vi "6) HTTP Info.vi"() -> ()   [LabVIEW 2020, in "VectoScratch.lvlib"]
uses:
  VectoScratch.lvlib
  Vecto/Node Config/Node Config.lvclass
  Vecto/Vecto/Vecto.lvclass
  Vecto/VectoService/VectoInfo.lvclass
  Vecto/ChannelService/ChannelService.lvclass
  Vecto/Group Config/Group Config.lvclass
  Vecto/Group Info.ctl
  VectoConfig/VectoConfig.lvlib
  Vecto/RemoteDataService/RemoteDataService.lvclass
  Vecto/Group DBL/Group DBL.lvclass
  Vecto/Group Data Type.ctl
  C:/dev/lv20CE/relink/lv-vecto/Vecto/Group/Group.lvclass
  C:/dev/lv20CE/relink/lv-vecto/Vecto/Group DBL/Group DBL.lvclass
  Vecto/Group STR/Group STR.lvclass
  C:/dev/lv20CE/relink/lv-vecto/Vecto/Group STR/Group STR.lvclass
  Vecto/Node Config/Discovery Info.ctl
  Vecto/Node Config/Node Info.ctl
  Vecto/Node Config/HTTP Server Info.ctl
  Vecto/Channel Init.ctl
  Vecto/IP Resolver/IP Resolver.lvclass
  Vecto/Connection Type.ctl
  Vecto/Vecto.lvlib
  Vecto/Connection Info.ctl
  Vecto/Vecto Info.ctl
  Vecto/proto/ServiceType/Enumeration.ctl
  Vecto/proto/ServiceType/ServiceType.lvlib
  Vecto/proto/Service/Data.ctl
  Vecto/proto/Service/Service.lvlib
  Vecto/proto/Discovery/Data.ctl
  Vecto/proto/Discovery/Discovery.lvlib
  Vecto/Publish Config.ctl
panel:
  in  "Strings":string[](array[string])=["alpha", "beta", "gamma", "delta"]
  in  "Publish Config":T1={"Address"="239.0.0.101", "Port"=36987}
  in  "Values":dbl[](array[slide])=[0.0, 0.0, 0.0, 0.0, 0.0, 0.0] scale=0.0..100.0
  in  "Bind Address":string="192.168.42.59"
  in  "ID":u32=1
  in  "Start":bool
  out "Discovery":T2[](array[typedef]) {"ip" format="%.0x"}
  in  "Discovery Address":string="239.0.0.50"
  in  "Discovery Port":u16=36986
  out "Vecto Info":T5
  in  "stop":bool
  in  "Node Name":string="Alpha"
  in  "HTTP Port":u16=36987
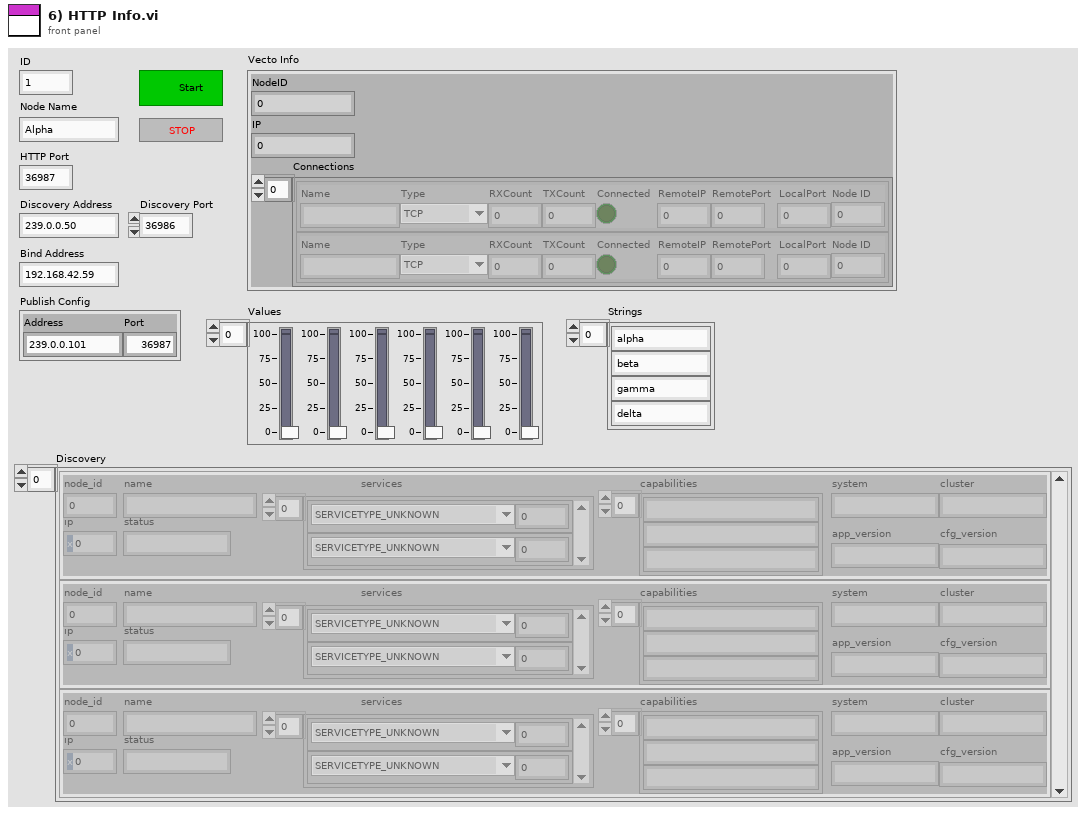
[diagram p1: front panel]
types:
  T1 = typedef "VectoConfig.lvlib/Publish Config.ctl" = cluster{"Address":string, "Port":u16}
  T2 = typedef "Discovery.lvlib/Data.ctl" = cluster{"node_id":u32, "name":string, "ip":u32, "status":string, "services":T3[], "capabilities":string[], "system":string, "cluster":string, "app_version":string, "cfg_version":string}
  T3 = typedef "Service.lvlib/Data.ctl" = cluster{"type":T4, "port":i32}
  T4 = typedef "ServiceType.lvlib/Enumeration.ctl" = enum16{"SERVICETYPE_UNKNOWN", "SERVICETYPE_TCPSERVER", "SERVICETYPE_HTTPSERVER"}
  T5 = typedef "Vecto.lvlib/Vecto Info.ctl" = cluster{"NodeID":i32, "IP":u32, "Connections":T6[]}
  T6 = typedef "Vecto.lvlib/Connection Info.ctl" = cluster{"Name":string, "Type":T7, "RXCount":i32, "TXCount":i32, "Connected":bool, "RemoteIP":u32, "RemotePort":u16, "LocalPort":u16, "Node ID":u32}
  T7 = typedef "Vecto.lvlib/Connection Type.ctl" = enum16{"TCP", "Telemetry", "Discovery", "HTTP"}
  T8 = typedef "VectoConfig.lvlib/Group Data Type.ctl" = enum16{"Double", "String", "Bool"}
  T9 = typedef "VectoConfig.lvlib/Group Info.ctl" = cluster{"System":string, "Cluster":string, "Node":string, "Task":string, "Name":string}
  T10 = typedef "VectoConfig.lvlib/HTTP Server Info.ctl" = cluster{"HTTP Port":u16, "Debug":bool}
  T11 = typedef "Discovery Info.ctl" = cluster{"Address":string, "Port":u16, "Interval S":dbl, "Bind Address":refnum<class "IP Resolver.lvclass">}
  T12 = typedef "VectoConfig.lvlib/Node Info.ctl" = cluster{"System":string, "Cluster":string, "Name":string, "ID":u32, "Capabilities":string[]}
  T13 = typedef "VectoConfig.lvlib/Channel Init.ctl" = cluster{"Name":string, "Resource":string, "Unit String":string}
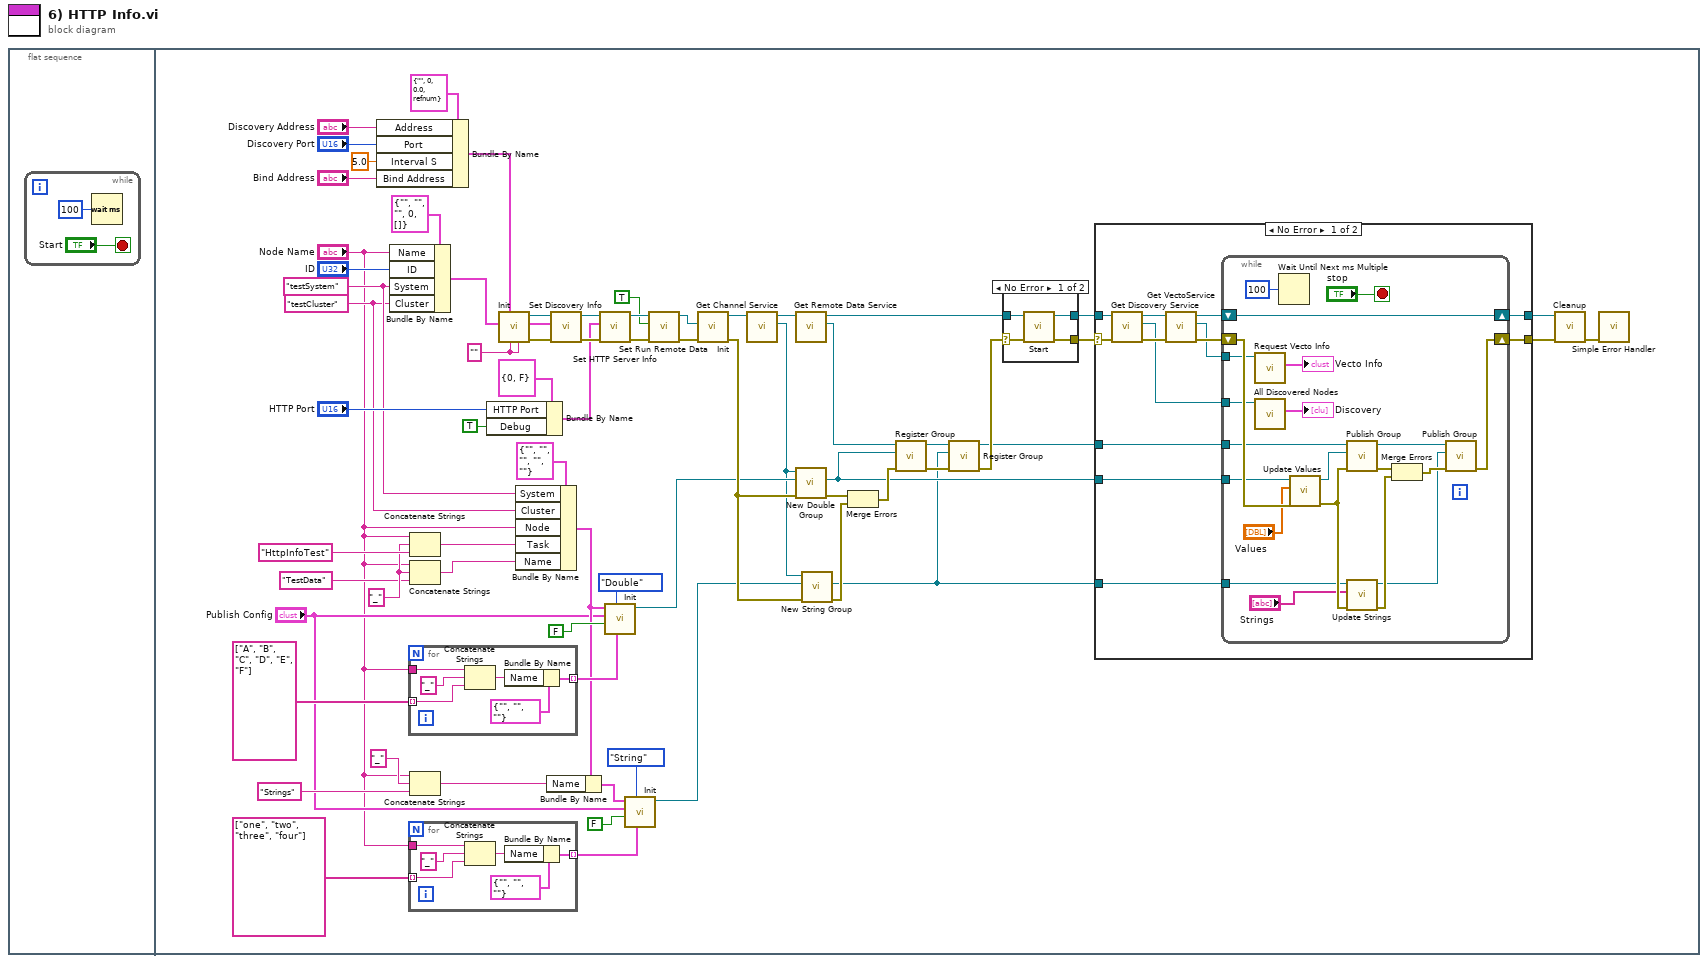
[diagram p0: block diagram]
diagram:
  n1 = flat-sequence {
    frame #0 {
      n2 = while {
        stop <- "Start" stop-if-true
        n3 = Wait (ms)(milliseconds to wait=u32 100) -> ()  [unwired: 1 out]
      }
    }
    frame #1 {
      w3 = "" ("Config Version")
      w30 = "_" ("string")
      w38 = "testCluster" ("System")
      w39 = "testSystem" ("System")
      n4 = Bundle By Name(cluster=T11 {"Address"="", "Port"=0, "Interval S"=0.0, "Bind Address"=refnum} ("Discovery Info"), "Address"="Discovery Address", "Port"="Discovery Port", "Interval S"=5.0, "Bind Address"="Bind Address") -> (w60:T11)
      n5 = Bundle By Name(cluster=T12 {"System"="", "Cluster"="", "Name"="", "ID"=0, "Capabilities"=[]} ("Node Info"), "Name"="Node Name", "ID"="ID", "System"=w39, "Cluster"=w38) -> (w56:T12)
      n6 = for {
        tunnel: string[] ["A", "B", "C", "D", "E", "F"] -> [w75] mode=indexing
        tunnel: "Node Name" -> [w74]
        tunnel: [w71] -> w26 mode=indexing
        n7 = Concatenate Strings(w74, "_" ("string"), w75) -> (w72:string)
        n8 = Bundle By Name(cluster=T13 {"Name"="", "Resource"="", "Unit String"=""} ("Channel Init"), "Name"=w72) -> (w71:T13)
      }
      n9 = for {
        tunnel: string[] ["one", "two", "three", "four"] -> [w123] mode=indexing
        tunnel: "Node Name" -> [w122]
        tunnel: [w119] -> w14 mode=indexing
        n10 = Concatenate Strings(w122, "_" ("string"), w123) -> (w120:string)
        n11 = Bundle By Name(cluster=T13 {"Name"="", "Resource"="", "Unit String"=""} ("Channel Init"), "Name"=w120) -> (w119:T13)
      }
      n12 = Concatenate Strings("Node Name", w30, "HttpInfoTest" ("Task")) -> (w31:string)
      n13 = Concatenate Strings("Node Name", w30, "TestData" ("Name")) -> (w28:string)
      n14 = Concatenate Strings("Node Name", "_" ("string"), "Strings" ("string")) -> (w21:string)
      n15 = Bundle By Name(cluster=T10 {"HTTP Port"=0, "Debug"=FALSE} ("HTTP Server Info"), "HTTP Port"="HTTP Port", "Debug"=TRUE) -> (w48:T10)
      n16 = call "Init.vi"("Config Hash"=w3, "Config Version"=w3, "Node Info"=w56) -> ("error out"=w63:errorcluster, "Node out"=w62:refnum<class "Node Config.lvclass">)  [unwired: 7 in]
      n17 = Bundle By Name(cluster=T9 {"System"="", "Cluster"="", "Node"="", "Task"="", "Name"=""} ("Group Info"), "System"=w39, "Cluster"=w38, "Node"="Node Name", "Task"=w31, "Name"=w28) -> (w24:T9)
      n18 = Bundle By Name(cluster=w24, "Name"=w21) -> (w20:T9)
      n19 = call "Set Discovery Info.vi"("error in (no error)"=w63, "Discovery Info"=w60, "Node in"=w62) -> ("error out"=w50:errorcluster, "Node out"=w51:refnum<class "Node Config.lvclass">)  [unwired: 7 in]
      n20 = call "Set HTTP Server Info.vi"("error in (no error)"=w50, "HTTP Server Info"=w48, "Node Config in"=w51) -> ("error out"=w45:errorcluster, "Node Config out"=w34:refnum<class "Node Config.lvclass">)  [unwired: 7 in]
      n21 = call "Init.vi"("Channels"=w26, "Group Data Type"=Group_Data_Type."Double", "Raw Values (T)"=FALSE, "Multicast Endpoint (None)"="Publish Config", "Group Info"=w24) -> ("Group Config out"=w42:refnum<class "Group Config.lvclass">)  [unwired: 5 in, 1 out]
      n22 = call "Init.vi"("Channels"=w14, "Group Data Type"=Group_Data_Type."String", "Raw Values (T)"=FALSE, "Multicast Endpoint (None)"="Publish Config", "Group Info"=w20) -> ("Group Config out"=w12:refnum<class "Group Config.lvclass">)  [unwired: 5 in, 1 out]
      n23 = call "Set Run Remote Data.vi"("error in (no error)"=w45, "Run Remote Data"=TRUE, "Node Config in"=w34) -> ("error out"=w35:errorcluster, "Node Config out"=w33:refnum<class "Node Config.lvclass">)  [unwired: 7 in]
      n24 = call "Init.vi"("error in (no error)"=w35, "Node"=w33) -> ("error out"=w70:errorcluster, "Vecto out"=w53:refnum<class "Vecto.lvclass">)  [unwired: 8 in]
      n25 = call "Get Channel Service.vi"("Vecto in"=w53) -> ("ChannelService"=w13:refnum<class "ChannelService.lvclass">, "Vecto out"=w52:refnum<class "Vecto.lvclass">)  [unwired: 8 in, 1 out]
      n26 = call "Get Remote Data Service.vi"("Vecto in"=w52) -> ("RemoteDataService"=w37:refnum<class "RemoteDataService.lvclass">, "Vecto out"=w44:refnum<class "Vecto.lvclass">)  [unwired: 8 in, 1 out]
      n27 = call "New Double Group.vi"("error in (no error)"=w70, "Group Config"=w42, "ChannelService in"=w13) -> ("error out"=w8:errorcluster, "Group"=w36:refnum<class "Group DBL.lvclass">)  [unwired: 6 in, 1 out]
      n28 = call "New String Group.vi"("error in (no error)"=w70, "Group Config"=w12, "ChannelService in"=w13) -> ("error out"=w69:errorcluster, "StringGroup"=w7:refnum<class "Group STR.lvclass">)  [unwired: 6 in, 1 out]
      n29 = Merge Errors(w8, w69) -> (w68:errorcluster)
      n30 = call "Register Group.vi"("error in (no error)"=w68, "Group"=w36, "RemoteDataService in"=w37) -> ("error out"=w67:errorcluster, "RemoteDataService out"=w11:refnum<class "RemoteDataService.lvclass">)  [unwired: 7 in]
      n31 = call "Register Group.vi"("error in (no error)"=w67, "Group"=w7, "RemoteDataService in"=w11) -> ("error out"=w10:errorcluster, "RemoteDataService out"=w9:refnum<class "RemoteDataService.lvclass">)  [unwired: 7 in]
      n32 = case shown="No Error" w10 {
        selector: w10 -> [w80 w82]
        tunnel: w44 -> [w79 w81]
        tunnel: [w78 w82] -> w66
        tunnel: [w77 w81] -> w65
        frame No Error {
          n33 = call "Start.vi"("error in (no error)"=w80, "Vecto in"=w79) -> ("error out"=w78:errorcluster, "Vecto out"=w77:refnum<class "Vecto.lvclass">)  [unwired: 8 in]
        }
        frame Error {
        }
      }
      n34 = case shown="No Error" w66 {
        selector: w66 -> [w91 w118]
        tunnel: [w94 w117] -> w5
        tunnel: [w93 w118] -> w4
        tunnel: w65 -> [w92 w117]
        tunnel: w9 -> [w85 _]
        tunnel: w36 -> [w84 _]
        tunnel: w7 -> [w83 _]
        frame No Error {
          n35 = call "Get Discovery Service.vi"("error in (no error)"=w91, "Vecto in"=w92) -> ("error out"=w95:errorcluster, "DiscoveryService"=w90:refnum<class "DiscoveryService.lvclass">, "Vecto out"=w89:refnum<class "Vecto.lvclass">)  [unwired: 7 in]
          n36 = call "Get VectoService.vi"("error in (no error)"=w95, "Vecto in"=w89) -> ("error out"=w87:errorcluster, "VectoService"=w86:refnum<class "VectoInfo.lvclass">, "Vecto out"=w88:refnum<class "Vecto.lvclass">)  [unwired: 7 in]
          n37 = while {
            shift-right: [w102] -> w93
            shift-left: w87 -> [w115]
            shift-right: [w113] -> w94
            shift-left: w88 -> [w113]
            tunnel: w86 -> [w111]
            tunnel: w90 -> [w109]
            tunnel: w85 -> [w105]
            tunnel: w84 -> [w107]
            tunnel: w83 -> [w101]
            stop <- "stop" stop-if-true
            n38 = call "Request Vecto Info.vi"("VectoService in"=w111) -> ("Vecto Info"=→"Vecto Info":T5)  [unwired: 8 in, 2 out]
            n39 = call "All Discovered Nodes.vi"("DiscoveryService in"=w109) -> ("Nodes"=→"Discovery":T2[])  [unwired: 8 in, 2 out]
            n40 = Wait Until Next ms Multiple(millisecond multiple=u32 100 ("milliseconds to wait")) -> ()  [unwired: 1 out]
            n41 = call "Update Values.vi"("error in (no error)"=w115, "Values"="Values", "Group in"=w107) -> ("error out"=w116:errorcluster, "Group out"=w104:refnum<class "Group DBL.lvclass">)  [unwired: 7 in]
            n42 = call "Publish Group.vi"("error in (no error)"=w116, "Group"=w104, "RemoteDataService in"=w105) -> ("error out"=w99:errorcluster, "RemoteDataService out"=w103:refnum<class "RemoteDataService.lvclass">)  [unwired: 7 in]
            n43 = call "Update Strings.vi"("error in (no error)"=w116, "Strings"="Strings", "StringGroup in"=w101) -> ("error out"=w98:errorcluster, "StringGroup out"=w96:refnum<class "Group STR.lvclass">)  [unwired: 7 in]
            n44 = Merge Errors(w99, w98) -> (w97:errorcluster)
            n45 = call "Publish Group.vi"("error in (no error)"=w97, "Group"=w96, "RemoteDataService in"=w103) -> ("error out"=w102:errorcluster)  [unwired: 7 in, 1 out]
          }
        }
        frame Error {
        }
      }
      n46 = call "Cleanup.vi"("error in (no error)"=w4, "Vecto in"=w5) -> ("error out"=w6:errorcluster)  [unwired: 9 in]
      n47 = call <vilib>:"Simple Error Handler.vi"("error in (no error)"=w6) -> ()  [unwired: 4 in, 5 out]
    }
  }
